vi "Populate Baudrates.vi"(8 "error in":errorcluster, 11 "UI Actor in":refnum<class "UI Actor.lvclass">) -> (0 "error out":errorcluster, 3 "UI Actor out":refnum<class "UI Actor.lvclass">)   [LabVIEW 2024, in "UI Actor.lvlib" / "UI Actor.lvclass"]
uses:
  UI Actor.lvclass
  UI Actor.lvclass/UI Actor.ctl
  Core/EDS/EDS.lvclass
  Controls/Supported Baudrates.ctl
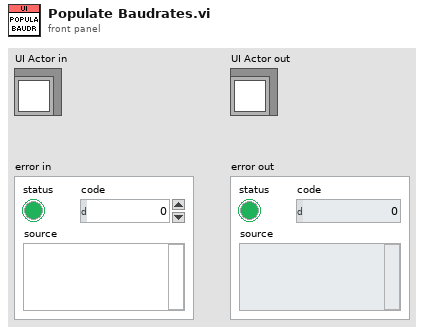
[diagram p1: front panel]
types:
  T1 = typedef "Supported Baudrates.ctl" = cluster{"10 kbps":bool, "20 kbps":bool, "50 kbps":bool, "125 kbps":bool, "250 kbps":bool, "500 kbps":bool, "800 kbps":bool, "1000 kbps":bool}
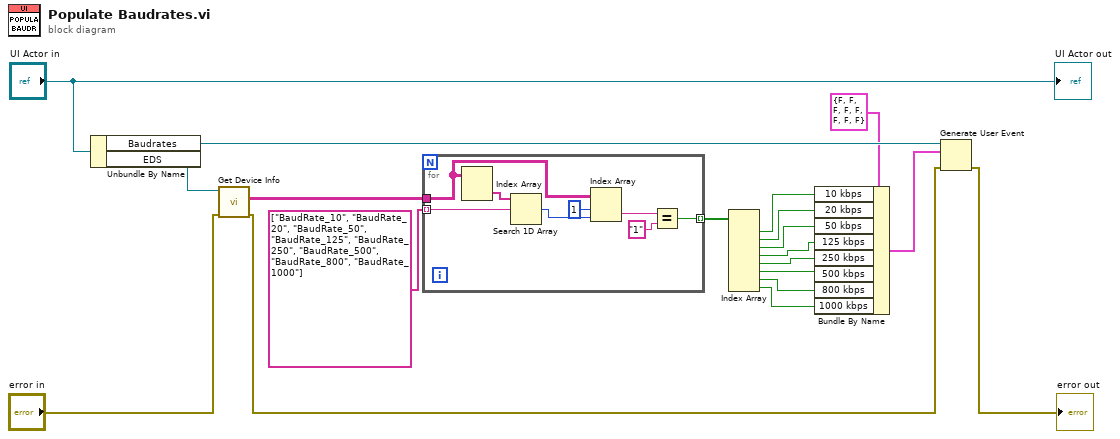
[diagram p0: block diagram]
diagram:
  n1 = Unbundle By Name("UI Actor in") -> ("Baudrates"=w18:refnum<user-event>, "EDS"=w19:refnum<class "EDS.lvclass">)
  n2 = call "Get Device Info.vi"("error in"="error in", "EDS in"=w19) -> ("error out"=w14:errorcluster, "Device Info"=w13:string[][])  [unwired: 7 in, 1 out]
  n3 = for {
    tunnel: string[] ["BaudRate_10", "BaudRate_20", "BaudRate_50", "BaudRate_125", "BaudRate_250", "BaudRate_500", "BaudRate_800", "BaudRate_1000"] -> [w27] mode=indexing
    tunnel: w13 -> [w25]
    tunnel: [w20] -> w9 mode=indexing
    n4 = Index Array(array=w25) -> (element=w26:string[])  [unwired: 2 in]
    n5 = Search 1D Array(1D array=w26, element=w27) -> (index of element=w24:i32)  [unwired: 1 in]
    n6 = Index Array(array=w25, index (row)=1, index (col)=w24) -> (element=w22:string)
    n7 = Equal?(x=w22, y="1") -> (x = y?=w20:bool)
  }
  n8 = Index Array(array=w9) -> (element #1=w8:bool, element #2=w7:bool, element #3=w6:bool, element #4=w5:bool, element #5=w4:bool, element #6=w3:bool, element #7=w2:bool, element #8=w1:bool)  [unwired: 8 in]
  n9 = Bundle By Name(cluster=T1 {"10 kbps"=FALSE, "20 kbps"=FALSE, "50 kbps"=FALSE, "125 kbps"=FALSE, "250 kbps"=FALSE, "500 kbps"=FALSE, "800 kbps"=FALSE, "1000 kbps"=FALSE} ("Baudrates"), "10 kbps"=w8, "20 kbps"=w7, "50 kbps"=w6, "125 kbps"=w5, "250 kbps"=w4, "500 kbps"=w3, "800 kbps"=w2, "1000 kbps"=w1) -> (w15:T1)
  n10 = Generate User Event(user event=w18, event data cluster=w15, error in=w14) -> (error out=→"error out":errorcluster)  [unwired: 1 in, 1 out]
  "UI Actor out" <- "UI Actor in"
